vi "Test_ParseErrorsFromAnswer.vi"(8 "error in (no error)":errorcluster) -> (0 "error out":errorcluster)   [LabVIEW 2020, in "horiba.test.lvlib"]
uses:
  horiba.test.lvlib
  Classes/Communicator/Communicator.lvclass
  <vilib>/addons/_JKI Toolkits/Caraya/classes/Assert/Assert Error.vi
  <vilib>/addons/_JKI Toolkits/Caraya/classes/Assert/Assert Not Error.vi
  <vilib>/addons/_JKI Toolkits/Caraya/classes/Assert/Assert Equal Value and Type_Variant.vi
panel:
  # "Connector Pane"
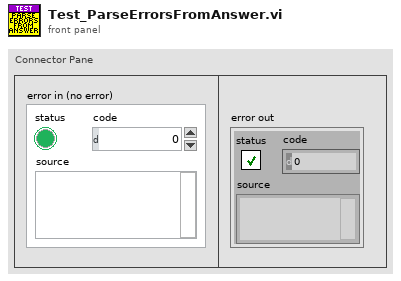
[diagram p1: front panel]
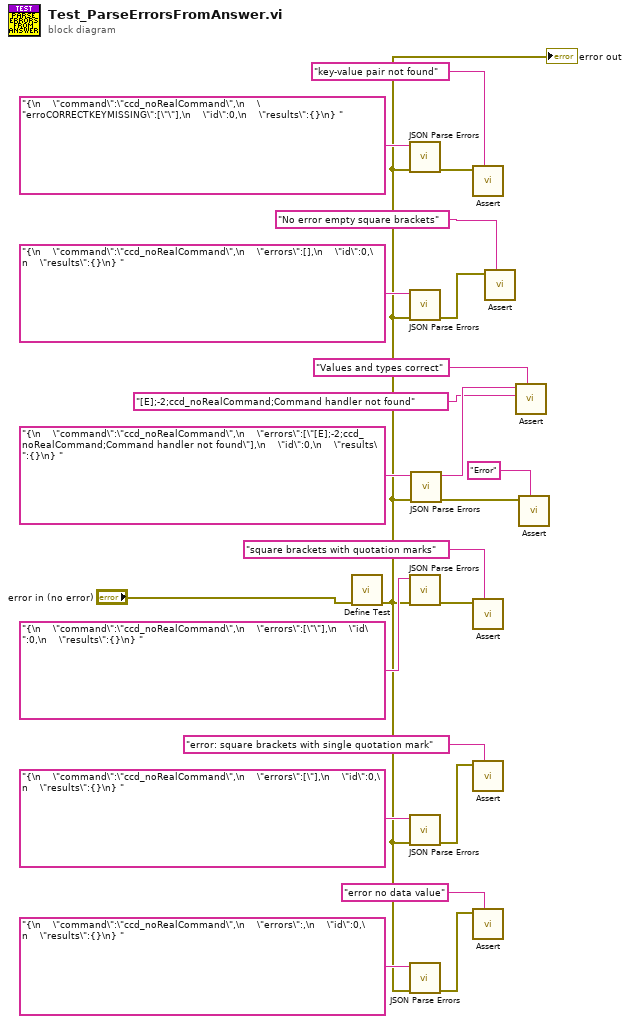
[diagram p0: block diagram]
diagram:
  n1 = call <vilib>:"Define Test.vi"("error in (no error)"="error in (no error)") -> ("error out"=w4:errorcluster)  [unwired: 9 in, 1 out]
  "error out" <- w4
  n2 = call "JSON Parse Errors.vi"("error in (no error)"=w4, "JSON command"="{\n    \"command\":\"ccd_noRealCommand\",\n    \"erroCORRECTKEYMISSING\":[\"\"],\n    \"id\":0,\n    \"results\":{}\n} ") -> ("error out"=w21:errorcluster)  [unwired: 7 in, 2 out]
  n3 = call "JSON Parse Errors.vi"("error in (no error)"=w4, "JSON command"="{\n    \"command\":\"ccd_noRealCommand\",\n    \"errors\":[],\n    \"id\":0,\n    \"results\":{}\n} ") -> ("error out"=w18:errorcluster)  [unwired: 7 in, 2 out]
  n4 = call "JSON Parse Errors.vi"("error in (no error)"=w4, "JSON command"="{\n    \"command\":\"ccd_noRealCommand\",\n    \"errors\":[\"\"],\n    \"id\":0,\n    \"results\":{}\n} ") -> ("error out"=w15:errorcluster)  [unwired: 7 in, 2 out]
  n5 = call "JSON Parse Errors.vi"("error in (no error)"=w4, "JSON command"="{\n    \"command\":\"ccd_noRealCommand\",\n    \"errors\":[\"],\n    \"id\":0,\n    \"results\":{}\n} ") -> ("error out"=w9:errorcluster)  [unwired: 7 in, 2 out]
  n6 = call "JSON Parse Errors.vi"("error in (no error)"=w4, "JSON command"="{\n    \"command\":\"ccd_noRealCommand\",\n    \"errors\":,\n    \"id\":0,\n    \"results\":{}\n} ") -> ("error out"=w12:errorcluster)  [unwired: 7 in, 2 out]
  n7 = call "JSON Parse Errors.vi"("error in (no error)"=w4, "JSON command"="{\n    \"command\":\"ccd_noRealCommand\",\n    \"errors\":[\"[E];-2;ccd_noRealCommand;Command handler not found\"],\n    \"id\":0,\n    \"results\":{}\n} ") -> ("error out"=w1:errorcluster, "error string (if existing)"=w3:string)  [unwired: 7 in, 1 out]
  n8 = call-poly <vilib>:"Assert.vi"("Label"="key-value pair not found" ("Label (VI Title)"), "Error?"=w21) -> ()  [unwired: 8 in, 2 out]
  n9 = call-poly <vilib>:"Assert.vi"("Label"="square brackets with quotation marks" ("Label (VI Title)"), "Error?"=w15) -> ()  [unwired: 8 in, 2 out]
  n10 = call-poly <vilib>:"Assert.vi"("Label"="error: square brackets with single quotation mark" ("Label (VI Title)"), "Error?"=w9) -> ()  [unwired: 8 in, 2 out]
  n11 = call-poly <vilib>:"Assert.vi"("Label"="error no data value" ("Label (VI Title)"), "Error?"=w12) -> ()  [unwired: 8 in, 2 out]
  n12 = call-poly <vilib>:"Assert.vi"("Label"="No error empty square brackets" ("Label (VI Title)"), "Not Error?"=w18) -> ()  [unwired: 8 in, 2 out]
  n13 = call-poly <vilib>:"Assert.vi"("Label"="Values and types correct" ("Label (VI Title)"), "Y"="[E];-2;ccd_noRealCommand;Command handler not found" ("error string (if existing) 7"), "X"=w3) -> ()  [unwired: 7 in, 2 out]
  n14 = call-poly <vilib>:"Assert.vi"("Label"="Error" ("Label (VI Title)"), "Error?"=w1) -> ()  [unwired: 8 in, 2 out]
